vi "Delete SV Libraries.vi"(8 "error in (no error)":errorcluster, 11 "SV B-M (Host) in":refnum<class "SV B-M (Host).lvclass">) -> (0 "error out":errorcluster, 3 "SV B-M (Host) out":refnum<class "SV B-M (Host).lvclass">)   [LabVIEW 2015, in "SV B-M (Host).lvclass"]
doc: "Delete all shared variable libraries used in this test from disk."
uses:
  SV B-M (Host).lvclass
  SV B-M (Host).lvclass/SV B-M (Host).ctl
  Listbox - In Progress.vi
  Listbox - Complete.vi
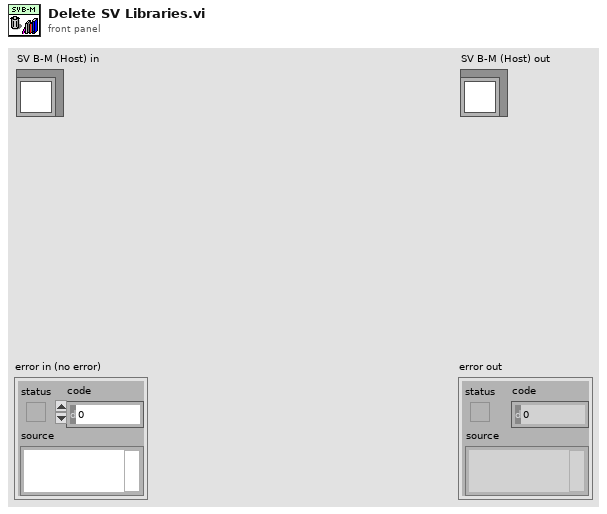
[diagram p1: front panel]
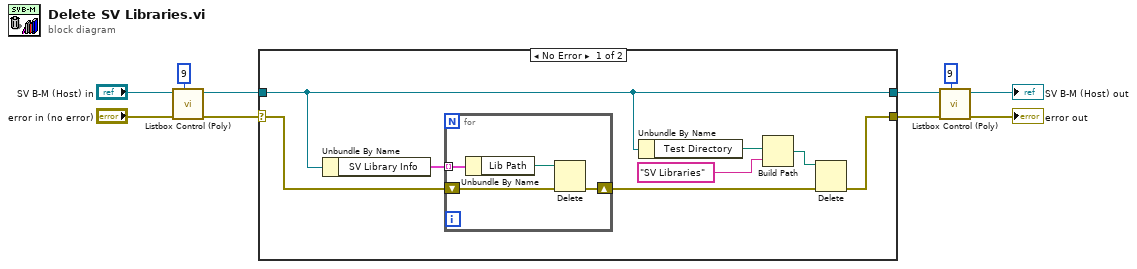
[diagram p0: block diagram]
diagram:
  n1 = call-poly "Listbox Control (Poly).vi"("Row to Update"=9, "error in (no error)"="error in (no error)", "SV B-M In"="SV B-M (Host) in") -> ("error out"=w7:errorcluster, "SV B-M Out"=w9:refnum<class "SV B-M (Host).lvclass">)  [unwired: 7 in]
  n2 = case shown="No Error" w7 {
    selector: w7 -> [w17 w24]
    tunnel: [w11 w24] -> w3
    tunnel: [w15 w23] -> w4
    tunnel: w9 -> [w15 w23]
    frame No Error {
      n3 = Unbundle By Name(w15) -> ("SV Library Info"=w18:cluster{"Lib Path":path, "Lib Size":u16}[])
      n4 = for {
        tunnel: w18 -> [w22] mode=indexing
        shift-right: [w19] -> w16
        shift-left: w17 -> [w21]
        n5 = Unbundle By Name(w22) -> ("Lib Path"=w20:path)
        n6 = Delete(path (use dialog)=w20, error in=w21) -> (error out=w19:errorcluster)  [unwired: 3 in, 2 out]
      }
      n7 = Unbundle By Name(w15) -> ("Test Directory"=w13:path)
      n8 = Build Path(base path=w13, name or relative path="SV Libraries") -> (appended path=w14:path)
      n9 = Delete(path (use dialog)=w14, error in=w16) -> (error out=w11:errorcluster)  [unwired: 3 in, 2 out]
    }
    frame Error {
    }
  }
  n10 = call-poly "Listbox Control (Poly).vi"("Row to Update"=9, "error in (no error)"=w3, "SV B-M In"=w4) -> ("error out"=→"error out":errorcluster, "SV B-M Out"=→"SV B-M (Host) out":refnum<class "SV B-M (Host).lvclass">)  [unwired: 7 in]
